vi "status_string_format.vi"(1 "log_file":path, 4 "marker":string, 5 "ip":string, 6 "eeg_device":T1, 7 "color":enum16{"Black", "Blue", "Red", "Time"}(ring), 8 "error in (no error)":errorcluster, 9 "index":i32, 10 "gui_strings":string[](array[string]), 11 "Message Queue":refnum<queue>) -> (0 "error out":errorcluster, 3 "dup Message Queue":refnum<queue>)   [LabVIEW 2013]
doc: "Edits the Color and format of the string of a GUI message, and put it in the GUI queue"
uses:
  queues/que_message_cluster.ctl
  type_def/device.ctl
  queues/que_enqueue_message_single.vi
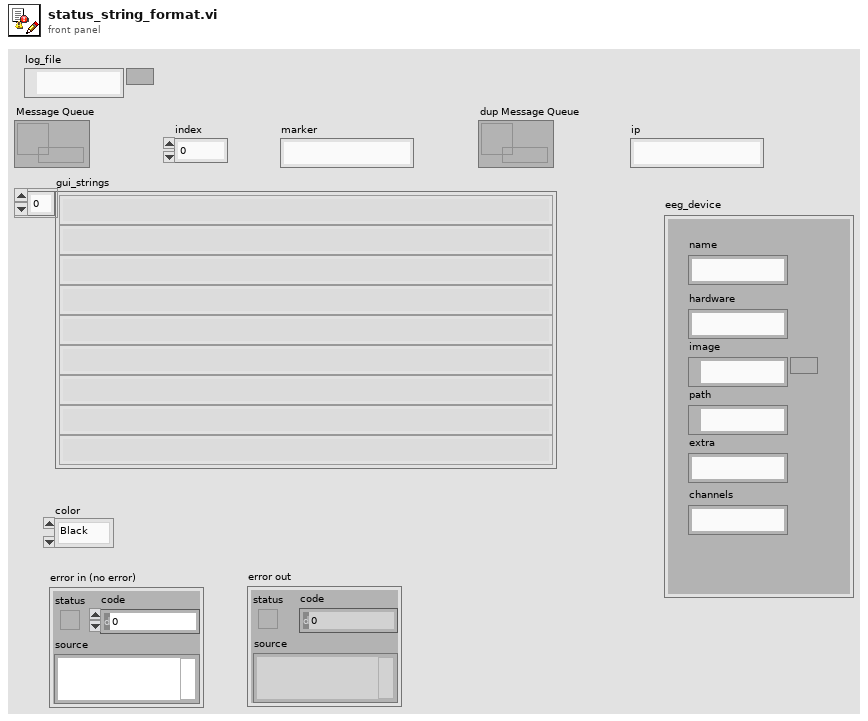
[diagram p1: front panel]
types:
  T1 = typedef "device.ctl" = cluster{"name":string, "hardware":string, "image":path, "path":path, "extra":string, "channels":string}
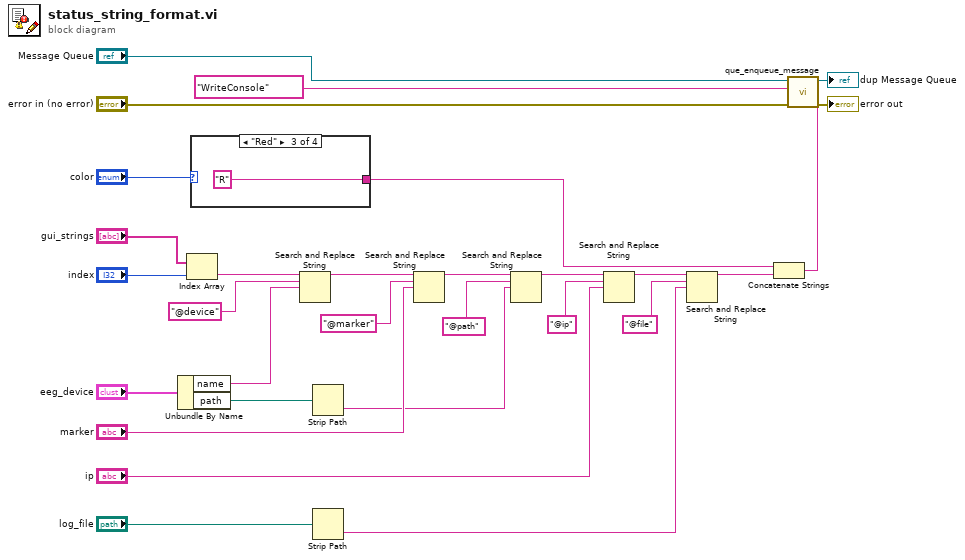
[diagram p0: block diagram]
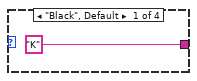
[diagram p2: hidden frame]
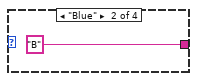
[diagram p3: hidden frame]
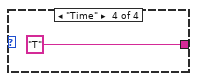
[diagram p4: hidden frame]
diagram:
  n1 = Unbundle By Name("eeg_device") -> ("name"=w22:string, "path"=w11:path)
  n2 = Index Array(array="gui_strings", index="index") -> (element=w25:string)
  n3 = case shown="\"Red\"" "color" {
    tunnel: ["K" "B" "R" "T"] -> w20
    frame "Black", Default {
    }
    frame "Blue" {
    }
    frame "Red" {
    }
    frame "Time" {
    }
  }
  n4 = Search and Replace String(input string=w25, search string="@device", replace string=w22) -> (result string=w18:string)  [unwired: 5 in, 3 out]
  n5 = Strip Path(path=w11) -> (name=w9:string)  [unwired: 1 out]
  n6 = Strip Path(path="log_file") -> (name=w3:string)  [unwired: 1 out]
  n7 = Search and Replace String(input string=w18, search string="@marker", replace string="marker") -> (result string=w12:string)  [unwired: 5 in, 3 out]
  n8 = Search and Replace String(input string=w12, search string="@path", replace string=w9) -> (result string=w8:string)  [unwired: 5 in, 3 out]
  n9 = Search and Replace String(input string=w8, search string="@ip", replace string="ip") -> (result string=w5:string)  [unwired: 5 in, 3 out]
  n10 = Search and Replace String(input string=w5, search string="@file", replace string=w3) -> (result string=w4:string)  [unwired: 5 in, 3 out]
  n11 = Concatenate Strings(w20, w4) -> (w19:string)
  n12 = call-poly "que_enqueue_message.vi"("error in (no error)"="error in (no error)", "Message Data"=w19, "Message"="WriteConsole", "Message Queue"="Message Queue") -> ("error out"=→"error out":errorcluster, "dup Message Queue"=→"dup Message Queue":refnum<queue>)  [unwired: 6 in]
